vi "Save DeviceID.vi"(8 "error in (no error)":errorcluster, 9 "DeviceID":T1, 10 "Parent Camera Node":refnum<k20>, 11 "DOM document in":refnum<k20>) -> (0 "error out":errorcluster)   [LabVIEW 2013]
uses:
  <resource>/objmgr/DOMUserDefRef.rc
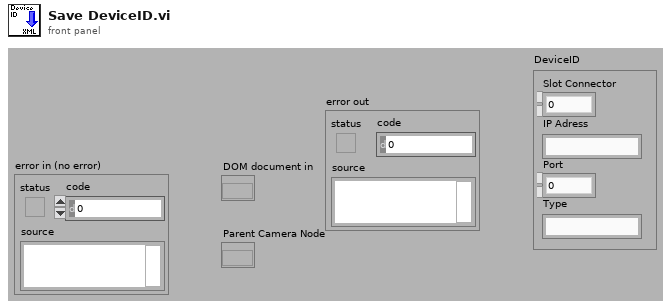
[diagram p1: front panel]
types:
  T1 = cluster{"Slot Connector":i32, "IP Adress":string, "Port":i32, "Type":string}
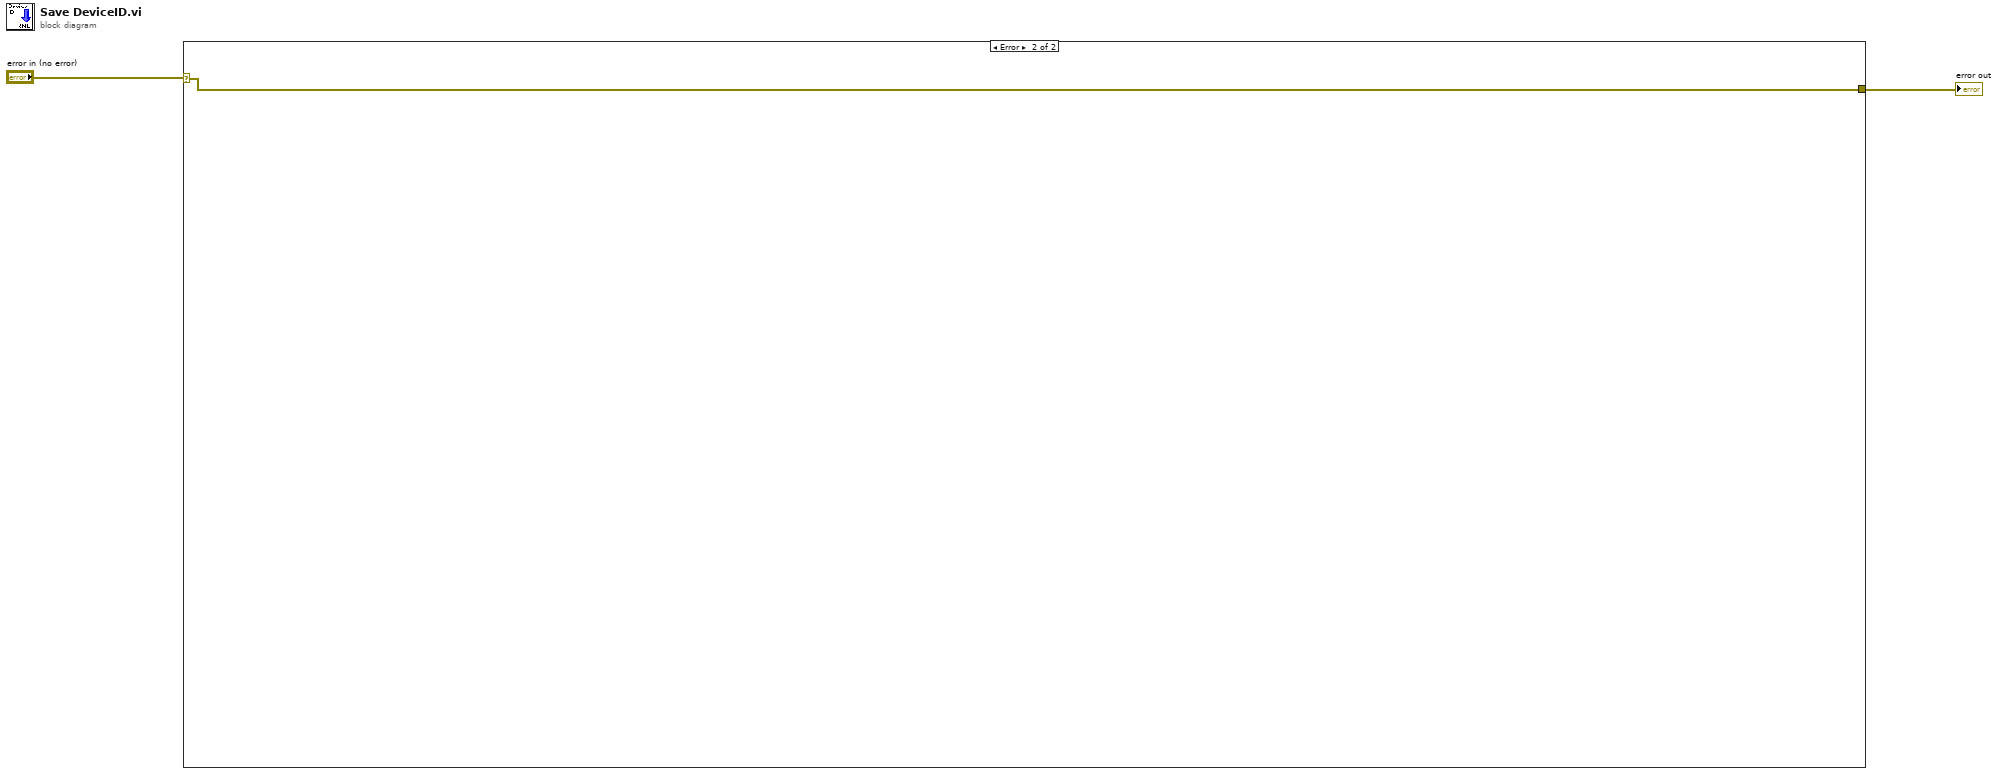
[diagram p0: block diagram]
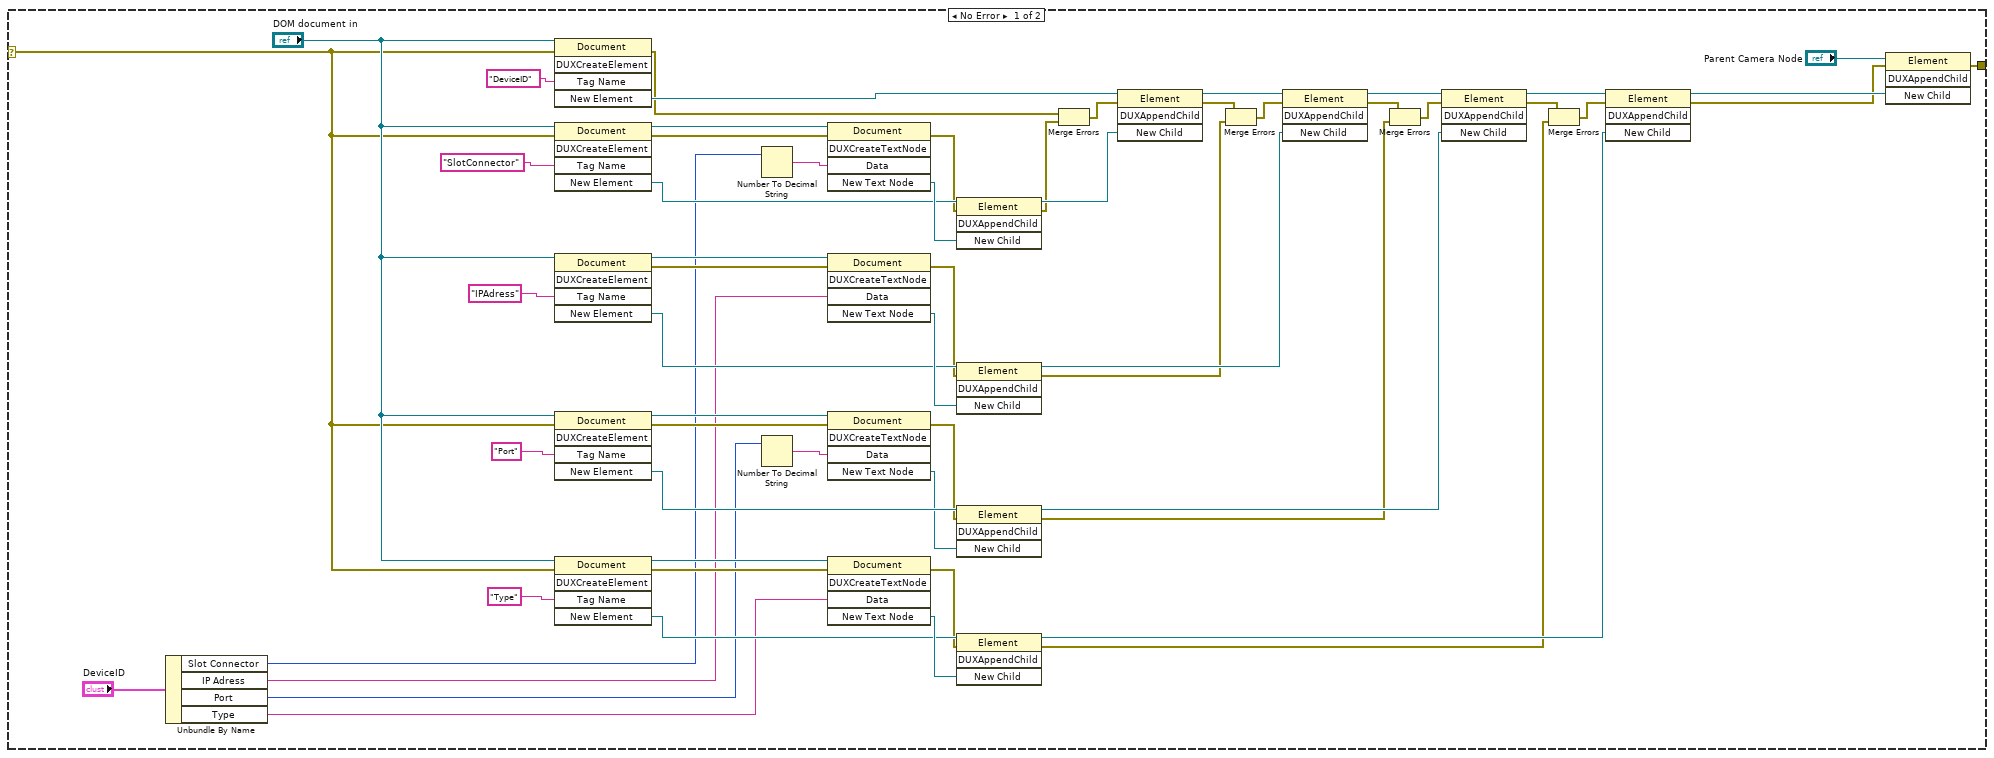
[diagram p2: hidden frame]
diagram:
  n1 = case shown="Error" "error in (no error)" {
    selector: "error in (no error)" -> [w3 w61]
    tunnel: [w11 w61] -> w2
    frame No Error {
      n2 = Unbundle By Name("DeviceID") -> ("Slot Connector"=w7:i32, "IP Adress"=w6:string, "Port"=w5:i32, "Type"=w4:string)
      n3 = invoke class="Document" method="DUXCreateElement"(reference="DOM document in", error in=w3, "Tag Name"="DeviceID") -> (error out=w22:errorcluster, "New Element"=w55:refnum<k20>)  [unwired: 2 in, 3 out]
      n4 = invoke class="Document" method="DUXCreateElement"(reference="DOM document in", error in=w3, "Tag Name"="SlotConnector") -> (reference out=w54:refnum<k20>, error out=w31:errorcluster, "New Element"=w50:refnum<k20>)  [unwired: 2 in, 2 out]
      n5 = invoke class="Document" method="DUXCreateElement"(reference="DOM document in", "Tag Name"="IPAdress") -> (reference out=w57:refnum<k20>, error out=w30:errorcluster, "New Element"=w52:refnum<k20>)  [unwired: 3 in, 2 out]
      n6 = invoke class="Document" method="DUXCreateElement"(reference="DOM document in", error in=w3, "Tag Name"="Port") -> (reference out=w44:refnum<k20>, error out=w29:errorcluster, "New Element"=w46:refnum<k20>)  [unwired: 2 in, 2 out]
      n7 = invoke class="Document" method="DUXCreateElement"(reference="DOM document in", error in=w3, "Tag Name"="Type") -> (reference out=w41:refnum<k20>, error out=w28:errorcluster, "New Element"=w39:refnum<k20>)  [unwired: 2 in, 2 out]
      n8 = Number To Decimal String(number=w7) -> (decimal integer string=w33:string)  [unwired: 1 in]
      n9 = Number To Decimal String(number=w5) -> (decimal integer string=w32:string)  [unwired: 1 in]
      n10 = invoke class="Document" method="DUXCreateTextNode"(reference=w54, error in=w31, "Data"=w33) -> (error out=w27:errorcluster, "New Text Node"=w51:refnum<k20>)  [unwired: 2 in, 3 out]
      n11 = invoke class="Document" method="DUXCreateTextNode"(reference=w57, error in=w30, "Data"=w6) -> (error out=w26:errorcluster, "New Text Node"=w53:refnum<k20>)  [unwired: 2 in, 3 out]
      n12 = invoke class="Document" method="DUXCreateTextNode"(reference=w44, error in=w29, "Data"=w32) -> (error out=w25:errorcluster, "New Text Node"=w45:refnum<k20>)  [unwired: 2 in, 3 out]
      n13 = invoke class="Document" method="DUXCreateTextNode"(reference=w41, error in=w28, "Data"=w4) -> (error out=w24:errorcluster, "New Text Node"=w40:refnum<k20>)  [unwired: 2 in, 3 out]
      n14 = invoke class="Element" method="DUXAppendChild"(reference=w50, error in=w27, "New Child"=w51) -> (reference out=w49:refnum<k20>, error out=w23:errorcluster)  [unwired: 1 in, 2 out]
      n15 = invoke class="Element" method="DUXAppendChild"(reference=w52, error in=w26, "New Child"=w53) -> (reference out=w48:refnum<k20>, error out=w18:errorcluster)  [unwired: 1 in, 2 out]
      n16 = invoke class="Element" method="DUXAppendChild"(reference=w46, error in=w25, "New Child"=w45) -> (reference out=w36:refnum<k20>, error out=w15:errorcluster)  [unwired: 1 in, 2 out]
      n17 = invoke class="Element" method="DUXAppendChild"(reference=w39, error in=w24, "New Child"=w40) -> (reference out=w35:refnum<k20>, error out=w12:errorcluster)  [unwired: 1 in, 2 out]
      n18 = Merge Errors(w22, w23) -> (w21:errorcluster)
      n19 = invoke class="Element" method="DUXAppendChild"(reference=w55, error in=w21, "New Child"=w49) -> (reference out=w56:refnum<k20>, error out=w19:errorcluster)  [unwired: 1 in, 2 out]
      n20 = Merge Errors(w19, w18) -> (w20:errorcluster)
      n21 = invoke class="Element" method="DUXAppendChild"(reference=w56, error in=w20, "New Child"=w48) -> (reference out=w38:refnum<k20>, error out=w16:errorcluster)  [unwired: 1 in, 2 out]
      n22 = Merge Errors(w16, w15) -> (w17:errorcluster)
      n23 = invoke class="Element" method="DUXAppendChild"(reference=w38, error in=w17, "New Child"=w36) -> (reference out=w37:refnum<k20>, error out=w13:errorcluster)  [unwired: 1 in, 2 out]
      n24 = Merge Errors(w13, w12) -> (w14:errorcluster)
      n25 = invoke class="Element" method="DUXAppendChild"(reference=w37, error in=w14, "New Child"=w35) -> (reference out=w10:refnum<k20>, error out=w9:errorcluster)  [unwired: 1 in, 2 out]
      n26 = invoke class="Element" method="DUXAppendChild"(reference="Parent Camera Node", error in=w9, "New Child"=w10) -> (error out=w11:errorcluster)  [unwired: 1 in, 3 out]
    }
    frame Error {
    }
  }
  "error out" <- w2
